vi "Init Pixel.vi"(10 "Coordinate":cdb) -> (3 "Pixel":refnum<class "Pixel.lvclass">)   [LabVIEW 2016, in "Pixel.lvclass"]
uses:
  Pixel.lvclass
  Pixel.lvclass/Pixel.ctl
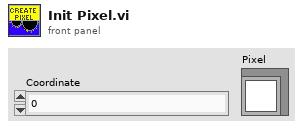
[diagram p1: front panel]
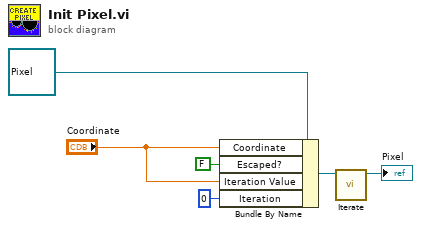
[diagram p0: block diagram]
diagram:
  n1 = Bundle By Name(cluster=refnum<class "Pixel.lvclass"> refnum ("Pixel.lvclass"), "Coordinate"="Coordinate", "Escaped?"=FALSE, "Iteration Value"="Coordinate", "Iteration"=u16 0) -> (w2:refnum<class "Pixel.lvclass">)
  n2 = call "Iterate.vi"("Pixel In"=w2) -> ("Pixel Outs"=→"Pixel":refnum<class "Pixel.lvclass">)  [unwired: 9 in, 1 out]
